vi "CRYResult Multi Language.vi"(10 "sOption":string, 11 "Verdict":bool) -> (3 "ASCII out":string)   [LabVIEW 2013]
uses:
  CRYMainGlobal.vi
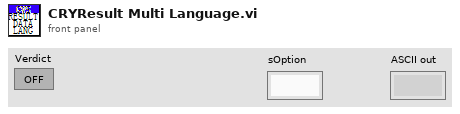
[diagram p1: front panel]
types:
  T1 = enum32{"English", "Chinese", "Korean", "Japanese", "Russian", "Chinese traditional"}
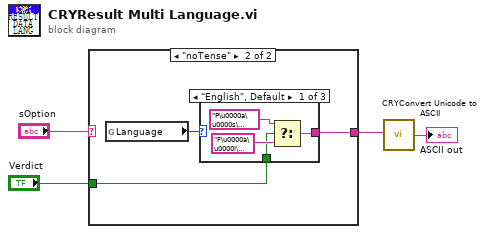
[diagram p0: block diagram]
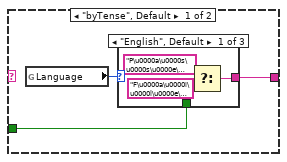
[diagram p2: hidden frame]
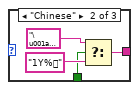
[diagram p3: hidden frame]
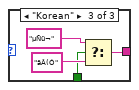
[diagram p4: hidden frame]
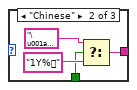
[diagram p5: hidden frame]
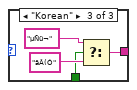
[diagram p6: hidden frame]
diagram:
  n1 = case shown="\"noTense\"" "sOption" {
    tunnel: [w6 w21] -> w4
    tunnel: "Verdict" -> [w5 w20]
    frame "byTense", Default {
      n2 = global read "CRYMainGlobal.vi" "Language"() -> (w7:T1)
      n3 = case shown="\"English\", Default" w7 {
        tunnel: [w9 w13 w17] -> w6
        tunnel: w5 -> [w8 w12 w16]
        frame "English", Default {
          n4 = Select(t="P\u0000a\u0000s\u0000s\u0000e\u0000d\u0000" ("Label.Text"), s=w8, f="F\u0000a\u0000i\u0000l\u0000e\u0000d\u0000" ("Label.Text")) -> (s? t:f=w9:string)
        }
        frame "Chinese" {
          n5 = Select(t="\u001aÇ" ("Label.Text"), s=w12, f="1Y%" ("Label.Text")) -> (s? t:f=w13:string)
        }
        frame "Korean" {
          n6 = Select(t="µÑü¬" ("Label.Text"), s=w16, f="äÂ(Ó" ("Label.Text")) -> (s? t:f=w17:string)
        }
      }
    }
    frame "noTense" {
      n7 = global read "CRYMainGlobal.vi" "Language"() -> (w22:T1)
      n8 = case shown="\"English\", Default" w22 {
        tunnel: [w24 w28 w32] -> w21
        tunnel: w20 -> [w23 w27 w31]
        frame "English", Default {
          n9 = Select(t="P\u0000a\u0000s\u0000s\u0000" ("Label.Text"), s=w23, f="F\u0000a\u0000i\u0000l\u0000" ("Label.Text")) -> (s? t:f=w24:string)
        }
        frame "Chinese" {
          n10 = Select(t="\u001aÇ" ("Label.Text"), s=w27, f="1Y%" ("Label.Text")) -> (s? t:f=w28:string)
        }
        frame "Korean" {
          n11 = Select(t="µÑü¬" ("Label.Text"), s=w31, f="äÂ(Ó" ("Label.Text")) -> (s? t:f=w32:string)
        }
      }
    }
  }
  n12 = call "CRYConvert Unicode to ASCII.vi"("Unicode"=w4) -> ("ASCII"=→"ASCII out":string)  [unwired: 4 in]
